vi "Command (read) - IS.vi"(7 "timeout ms (100)":i32=100, 8 "error in (no error)":errorcluster, 10 "IP":string, 11 "connection ID in":refnum<k16>) -> (0 "error out":errorcluster, 2 "Input Status":string, 3 "connection ID out":refnum<k16>)   [LabVIEW 2016, in "SMD-7615.lvlib" / "eSCL.lvlib"]
doc: "IS - Input Status\nRequests immediate status of all drive inputs. A closed input is represented by a “0” (zero), and an open input is represented by a “1” (one). Unused positions in the response are represented by “0” (zero)."
uses:
  eSCL.lvlib
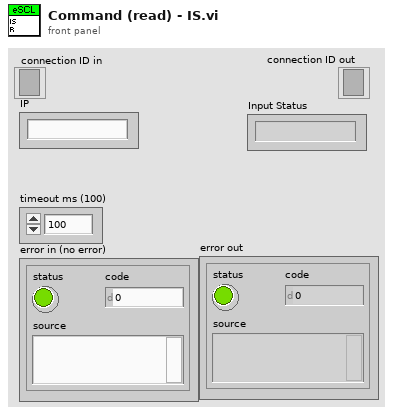
[diagram p1: front panel]
types:
  T1 = typedef "SMD-7615.lvlib/eSCL.lvlib/UDP Received Data.ctl" = cluster{"Received String":string, "eSCL Cmd":string, "Data":string}
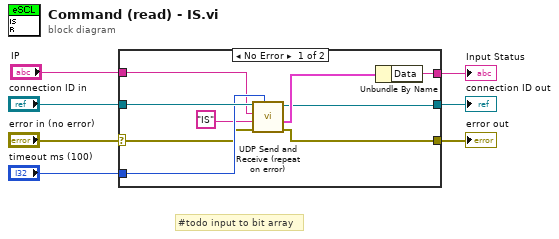
[diagram p0: block diagram]
diagram:
  # "#todo input to bit array"
  n1 = case shown="No Error" "error in (no error)" {
    selector: "error in (no error)" -> [w13 w17]
    tunnel: "connection ID in" -> [w15 w18]
    tunnel: [w8 w18] -> w5
    tunnel: [w9 w17] -> w4
    tunnel: "IP" -> [w11 _]
    tunnel: "timeout ms (100)" -> [w14 _]
    tunnel: [w16 _] -> w1
    frame No Error {
      n2 = call "UDP Send and Receive (repeat on error).vi"("timeout ms (100)"=w14, "error in (no error)"=w13, "Data"="IS", "IP"=w11, "connection ID in"=w15) -> ("error out"=w9:errorcluster, "Received Data"=w10:T1, "connection ID out"=w8:refnum<k16>)  [unwired: 3 in, 1 out]
      n3 = Unbundle By Name(w10) -> ("Data"=w16:string)
    }
    frame Error {
    }
  }
  "connection ID out" <- w5
  "error out" <- w4
  "Input Status" <- w1
